vi "Init.vi"(8 "error in (no error)":errorcluster, 11 "Crusher in":refnum<class "Crusher.lvclass">) -> (0 "error out":errorcluster, 3 "Crusher out":refnum<class "Crusher.lvclass">)   [LabVIEW 2019, in "Crusher.lvlib" / "Crusher.lvclass"]
uses:
  Crusher.lvclass
  Plugin Interfaces/Effect Interface/Effect Interface.lvlibp/Plugin Interfaces/Effect Interface/Effect Interface Class/Effect Interface.lvclass
  Plugin Interfaces/Effect Interface/Effect Interface.lvlibp/Libraries/Audio Processing/Value Properties.ctl
  Plugin Interfaces/Effect Interface/Effect Interface.lvlibp/Libraries/Audio Processing/Audio Processing.lvlib
  Plugin Interfaces/Effect Interface/Effect Interface.lvlibp/Libraries/Audio Processing/Value Cluster.ctl
  C:/github/dataflowg/dataflow-dj/src/Plugin Interfaces/Effect Interface/Effect Interface.lvlibp/Plugin Interfaces/Effect Interface/Effect Interface Class/Effect Interface.lvclass
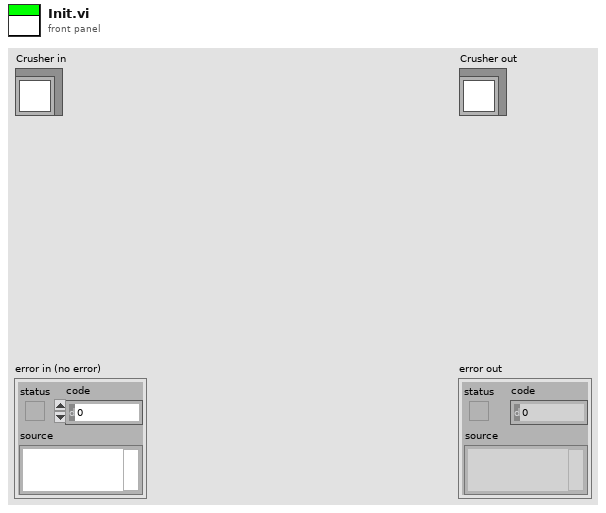
[diagram p1: front panel]
types:
  T1 = typedef "Effect Interface.lvlibp/Audio Processing.lvlib/Value Cluster.ctl" = cluster{"Value":dbl, "Properties":T2}
  T2 = typedef "Effect Interface.lvlibp/Audio Processing.lvlib/Value Properties.ctl" = cluster{"Lower":dbl, "Upper":dbl, "Default":dbl, "Increment":dbl}
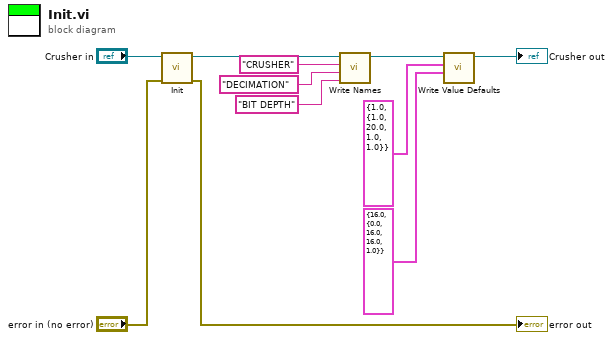
[diagram p0: block diagram]
diagram:
  n1 = call-parent "Init.vi"("error in (no error)"="error in (no error)", "Effect Interface in"="Crusher in") -> ("error out"=→"error out":errorcluster, "Effect Interface out"=w2:refnum<class "Crusher.lvclass">)  [unwired: 8 in]
  n2 = call "Write Names.vi"("Value2 Name"="BIT DEPTH" ("Value1 Name"), "Value1 Name"="DECIMATION", "Effect Name"="CRUSHER", "Effect Interface in"=w2) -> ("Effect Interface out"=w6:refnum<class "Crusher.lvclass">)  [unwired: 7 in]
  n3 = call "Write Value Defaults.vi"("Value2"=T1 {"Value"=16.0, "Properties"={"Lower"=0.0, "Upper"=16.0, "Default"=16.0, "Increment"=1.0}} ("Value1"), "Value1"=T1 {"Value"=1.0, "Properties"={"Lower"=1.0, "Upper"=20.0, "Default"=1.0, "Increment"=1.0}}, "Effect Interface in"=w6) -> ("Effect Interface out"=→"Crusher out":refnum<class "Crusher.lvclass">)  [unwired: 8 in]
